vi "Comm Command Engine.vi"(6 "Update Rate":u32=10, 8 "error in (no error)":errorcluster, 10 "Comm.lvclass":refnum<class "VeriStand Comm.lvclass">, 11 "Process":refnum<class "Process.lvclass">) -> (0 "error out":errorcluster)   [LabVIEW 2015, in "NI VeriStand Addon Network Comm.lvlib" / "VeriStand Comm.lvclass"]
uses:
  VeriStand Comm.lvclass
  <vilib>/NI/NI VeriStand Inline Async API/_VS Inline Async API/Process/Process.lvclass
  VeriStand Comm.lvclass/VeriStand Comm.ctl
  <vilib>/NI/STM/Connection Manager/TCP/TCP Connection Method.ctl
  <vilib>/NI/STM/TCP/TCP Read Options.ctl
  Shared/_Types/Comm Message.ctl
  <vilib>/NI/STM/TCP/TCP Write Options.ctl
  <vilib>/NI/NI VeriStand Inline Async API/_VS Inline Async API/Process/Process.lvclass/Process.ctl
  <vilib>/NI/STM/TCP/Get Connection Reference (TCP).vi
  <vilib>/NI/AMC/Create Single Message.vi
  <vilib>/NI/AMC/Update Message Routing Info.vi
  <vilib>/NI/Tools/Keyed Array/Map String.vi
  <vilib>/NI/AMC/Read Termination Message.vi
  <vilib>/NI/NI VeriStand Inline Async API/_VS Inline Async API/Error Handling Process/SubVIs/Error.ConvertArray.vi
  <vilib>/NI/Tools/String/Get Case Matching.vi
  <vilib>/NI/STM/TCP/Write Message (TCP).vi
  <vilib>/NI/AMC/Globals.vi
  <vilib>/NI/AMC/Send Message.vi
  Shared/Comm Constants.vi
  <vilib>/NI/STM/TCP/Read Message (TCP).vi
  <vilib>/NI Veristand/Custom Device Tools/Custom Device Utility Library/Custom Device Utility Library.lvlib
  <vilib>/NI/Tools/Keyed Array/Tools_KeyedArray.lvlib
  <vilib>/NI/AMC/AMC.lvlib
  <vilib>/NI/STM/NI STM.lvlib
  Shared/NI VeriStand Addon Network Comm Shared.lvlib
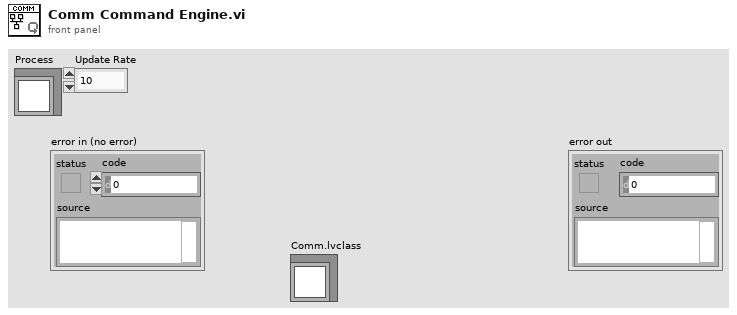
[diagram p1: front panel]
types:
  T1 = typedef "AMC.lvlib/Message Queue.ctl" = refnum<queue>
  T2 = typedef "TCP Connection Manager Reference.ctl" = refnum<data-value>
  T3 = typedef "NI STM.lvlib/TCP Connection Method.ctl" = enum16{"Initialize", "Add Connection", "Set Properties", "Get Connection(s)", "Remove Connection", "Remove All Connections", "Get Connection Count"}
  T4 = typedef "NI STM.lvlib/TCP Read Options.ctl" = cluster{"ignore timeout error":bool, "timeout ms (1000)":i32}
  T5 = typedef "NI VeriStand Addon Network Comm Shared.lvlib/Comm Message.ctl" = cluster{"Timeout":u32, "Resp?":bool, "data":string}
  T6 = typedef "NI STM.lvlib/TCP Write Options.ctl" = cluster{"ignore timeout error":bool, "timeout ms (1000)":i32}
  T7 = typedef "NI STM.lvlib/TCP Connection Info.ctl" = cluster{"connection ID":refnum<k5>, "meta data":T8[]}
  T8 = typedef "NI STM.lvlib/MetaDataElement.ctl" = string
  T9 = typedef "Tools_KeyedArray.lvlib/KeyedArray.ctl" = cluster{"keys":string[], "values":string[]}
  T10 = typedef "NI STM.lvlib/TCP Connection Properties.ctl" = cluster{"Name":string, "Address":string, "Custom":string}
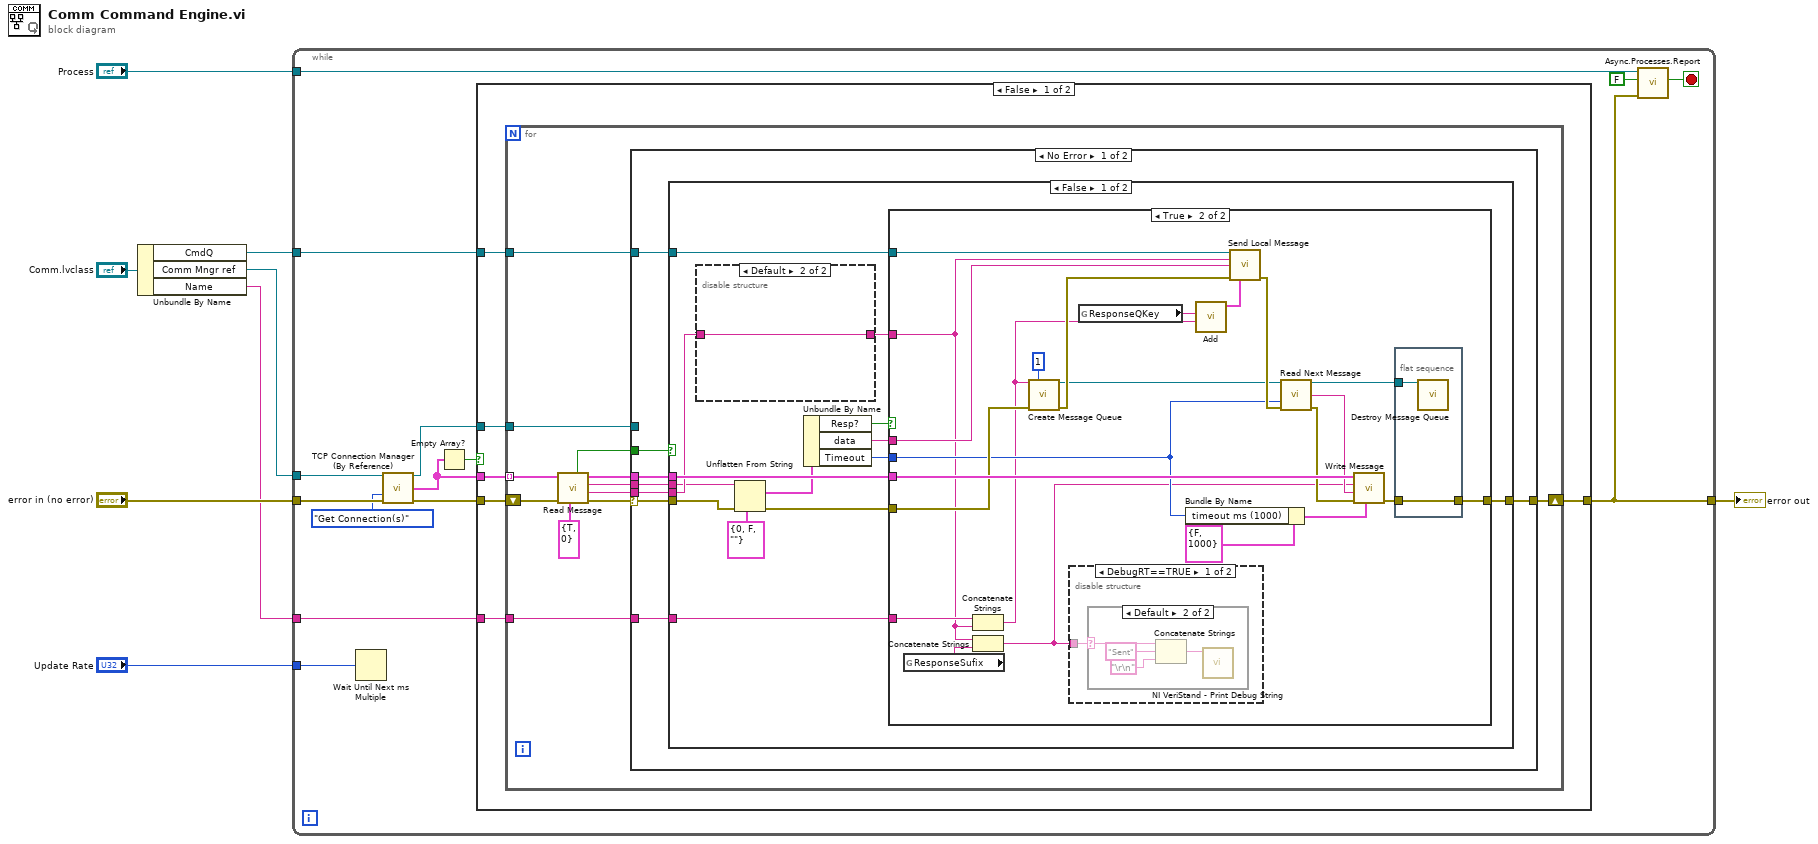
[diagram p0: block diagram]
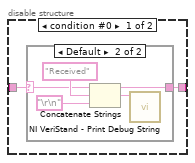
[diagram p2: hidden frame]
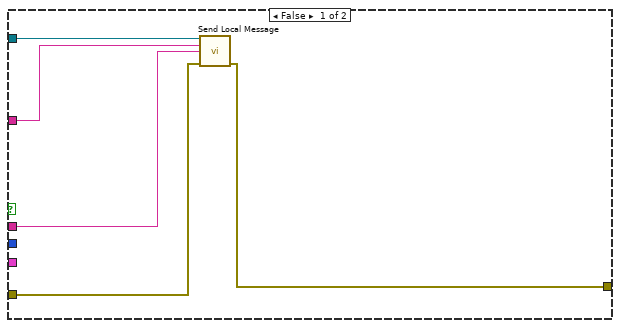
[diagram p4: hidden frame]
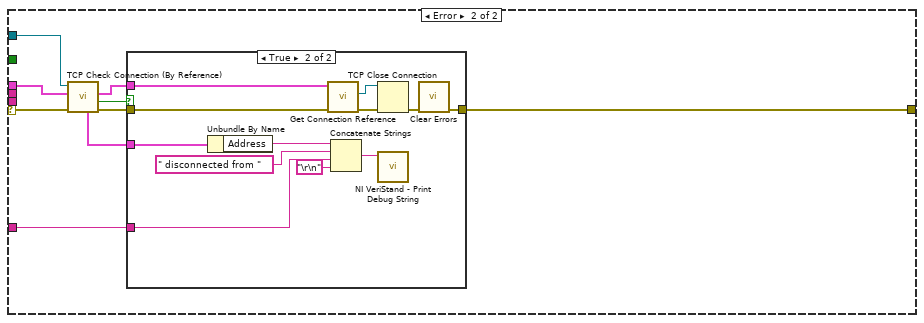
[diagram p8: hidden frame]
diagram:
  n1 = Unbundle By Name("Comm.lvclass") -> ("CmdQ"=w3:T1, "Comm Mngr ref"=w7:T2, "Name"=w4:string)
  n2 = while {
    tunnel: "error in (no error)" -> [w20]
    tunnel: [w11] -> w5
    tunnel: w7 -> [w17]
    tunnel: "Process" -> [w14]
    tunnel: w4 -> [w16]
    tunnel: w3 -> [w15]
    tunnel: "Update Rate" -> [w9]
    stop <- w12 stop-if-true
    n3 = Wait Until Next ms Multiple(millisecond multiple=w9) -> ()  [unwired: 1 out]
    n4 = call <vilib>:"TCP Connection Manager (By Reference).vi"("connection manager ref in"=w17, "method"=TCP_Connection_Method."Get Connection(s)", "error in"=w20) -> ("connection manager ref out"=w18:T2, "all connections"=w21:T7[], "error out"=w19:errorcluster)  [unwired: 6 in, 4 out]
    n5 = Empty Array?(array=w21) -> (empty?=w22:bool)
    n6 = case shown="False" w22 {
      tunnel: w21 -> [w28 _]
      tunnel: w19 -> [w24 w129]
      tunnel: w18 -> [w27 _]
      tunnel: [w26 w129] -> w11
      tunnel: w16 -> [w25 _]
      tunnel: w15 -> [w23 _]
      frame False {
        n7 = for {
          tunnel: w28 -> [w35] mode=indexing
          tunnel: w27 -> [w40]
          shift-right: [w39] -> w26
          shift-left: w24 -> [w37]
          tunnel: w25 -> [w38]
          tunnel: w23 -> [w30]
          n8 = call-poly <vilib>:"Read Message.vi"("options"=T4 {"ignore timeout error"=TRUE, "timeout ms (1000)"=0}, "error in"=w37, "connection info in"=w35) -> ("error out"=w36:errorcluster, "name"=w32:T8, "data string"=w33:string, "connection info out"=w34:T7, "timed out?"=w31:bool)  [unwired: 3 in, 1 out]
          n9 = case shown="No Error" w36 {
            selector: w36 -> [w48 w110]
            tunnel: w40 -> [_ w112]
            tunnel: w34 -> [w41 w111]
            tunnel: [w47 w109] -> w39
            tunnel: w38 -> [w42 w108]
            tunnel: w33 -> [w46 _]
            tunnel: w32 -> [w45 _]
            tunnel: w31 -> [w44 _]
            tunnel: w30 -> [w43 _]
            frame No Error {
              n10 = case shown="False" w44 {
                tunnel: w48 -> [w51 w106]
                tunnel: [w62 w106] -> w47
                tunnel: w46 -> [w50 _]
                tunnel: w45 -> [w58 _]
                tunnel: w43 -> [w61 _]
                tunnel: w42 -> [w60 _]
                tunnel: w41 -> [w59 _]
                frame False {
                  n11 = disable-structure shown="Default" {
                    disable-tunnel: w58 -> [w64 w70]
                    disable-tunnel: [w63 w70] -> w49
                    frame condition #0 {
                      n12 = case shown="Default" w64 {
                        selector: w64 -> [w65 w66]
                        tunnel: [w65 w66] -> w63
                        frame "" {
                        }
                        frame Default {
                          n13 = Concatenate Strings(w66, "Received" ("string"), "\r\n") -> (w69:string)
                          n14 = call <vilib>:"NI VeriStand - Print Debug String.vi"("Message"=w69) -> ()  [unwired: 10 in, 1 out]
                        }
                      }
                    }
                    frame condition #1 (active) {
                    }
                  }
                  n15 = Unflatten From String(type=T5 {"Timeout"=0, "Resp?"=FALSE, "data"=""}, binary string=w50, error in (no error)=w51) -> (value=w55:T5, error out=w57:errorcluster)  [unwired: 2 in, 1 out]
                  n16 = Unbundle By Name(w55) -> ("Resp?"=w52:bool, "data"=w54:string, "Timeout"=w53:u32)
                  n17 = case shown="True" w52 {
                    tunnel: [w72 w79] -> w62
                    tunnel: w61 -> [w75 w98]
                    tunnel: w60 -> [_ w97]
                    tunnel: w59 -> [_ w96]
                    tunnel: w57 -> [w73 w92]
                    tunnel: w54 -> [w74 w91]
                    tunnel: w53 -> [_ w88]
                    tunnel: w49 -> [w71 w78]
                    frame False {
                      n18 = call <vilib>:"Send Local Message.vi"("message queue in"=w75, "message name"=w71, "message value"=w74, "error in"=w73) -> ("error out"=w72:errorcluster)  [unwired: 9 in, 2 out]
                    }
                    frame True {
                      n19 = global read "Comm Constants.vi" "ResponseSufix"() -> (w76:string)
                      n20 = Concatenate Strings(w97, w78) -> (w84:string)
                      n21 = Concatenate Strings(w78, w76) -> (w85:string)
                      n22 = call <vilib>:"Create Message Queue.vi"("message queue name"=w84, "max queue size (-1, unlimited)"=1, "error in"=w92) -> ("message queue out"=w93:T1, "error out"=w95:errorcluster)  [unwired: 11 in]
                      n23 = disable-structure shown="DebugRT==TRUE" {
                        disable-tunnel: w85 -> [w99 _]
                        frame condition #0 {
                          n24 = case shown="Default" w99 {
                            selector: w99 -> [_ w101]
                            frame "" {
                            }
                            frame Default {
                              n25 = Concatenate Strings(w101, "Sent" ("string"), "\r\n") -> (w103:string)
                              n26 = call <vilib>:"NI VeriStand - Print Debug String.vi"("Message"=w103) -> ()  [unwired: 10 in, 1 out]
                            }
                          }
                        }
                        frame condition #1 (active) {
                        }
                      }
                      n27 = global read "Comm Constants.vi" "ResponseQKey"() -> (w77:string)
                      n28 = Bundle By Name(cluster=T6 {"ignore timeout error"=FALSE, "timeout ms (1000)"=1000} ("options"), "timeout ms (1000)"=w88) -> (w80:T6)
                      n29 = call <vilib>:"Add.vi"("value"=w84, "key"=w77) -> ("array out"=w83:T9)  [unwired: 3 in, 2 out]
                      n30 = call <vilib>:"Send Local Message.vi"("message queue in"=w98, "message name"=w78, "message value"=w91, "error in"=w95, "message attributes"=w83) -> ("error out"=w94:errorcluster)  [unwired: 8 in, 2 out]
                      n31 = call <vilib>:"Read Next Message.vi"("message queue in"=w93, "timeout (1 ms)"=w88, "error in"=w94) -> ("message queue out"=w87:T1, "message value"=w89:string, "error out"=w90:errorcluster)  [unwired: 5 in, 5 out]
                      n32 = call-poly <vilib>:"Write Message.vi"("options"=w80, "error in"=w90, "data"=w89, "name"=w85, "connection info in"=w96) -> ("error out"=w86:errorcluster)  [unwired: 5 in, 1 out]
                      n33 = flat-sequence {
                        tunnel: w87 -> [w105]
                        tunnel: w86 -> [w104]
                        tunnel: [w104] -> w79
                        frame #0 {
                          n34 = call <vilib>:"Destroy Message Queue.vi"("message queue in"=w105) -> ()  [unwired: 12 in, 3 out]
                        }
                      }
                    }
                  }
                }
                frame True {
                }
              }
            }
            frame Error {
              n35 = call <vilib>:"TCP Check Connection (By Reference).vi"("error in"=w110, "connection in"=w111, "connection manager ref in"=w112) -> ("error out"=w115:errorcluster, "disconnected?"=w113:bool, "connection out"=w114:T7, "properties out"=w107:T10)  [unwired: 4 in, 1 out]
              n36 = case shown="True" w113 {
                tunnel: [w116 w125] -> w109
                tunnel: w115 -> [w116 w128]
                tunnel: w114 -> [_ w123]
                tunnel: w108 -> [_ w118]
                tunnel: w107 -> [_ w117]
                frame False {
                }
                frame True {
                  n37 = Unbundle By Name(w117) -> ("Address"=w120:string)
                  n38 = call-poly <vilib>:"Get Connection Reference.vi"("error in"=w128, "connection info in"=w123) -> ("error out"=w127:errorcluster, "connection ID out"=w126:refnum<k5>)  [unwired: 7 in, 1 out]
                  n39 = Concatenate Strings(w120, " disconnected from " ("string"), w118, "\r\n") -> (w122:string)
                  n40 = TCP Close Connection(connection ID=w126, error in (no error)=w127) -> (error out=w124:errorcluster)  [unwired: 1 in, 1 out]
                  n41 = call <vilib>:"NI VeriStand - Print Debug String.vi"("Message"=w122) -> ()  [unwired: 10 in, 1 out]
                  n42 = call <vilib>:"Clear Errors.vi"("error in (no error)"=w124) -> ("error out"=w125:errorcluster)  [unwired: 5 in, 1 out]
                }
              }
            }
          }
        }
      }
      frame True {
      }
    }
    n43 = call <vilib>:"Async.Processes.Report.vi"("Error"=w11, "Stop Async on Error?"=FALSE ("Stop on Error?"), "Process in"=w14) -> ("Stop"=w12:bool)  [unwired: 7 in, 1 out]
  }
  "error out" <- w5
